vi "VisionMain.vi"(6 "Generated Distance Array":dbl[][](array[numeric]), 7 "Database Total Points":i32, 8 "Y Center":dbl, 9 "X Center":dbl, 10 "Original Plots":T1(array[cluster]), 11 "Plots Captured":T1(array[cluster])) -> (1 "alpha":dbl, 2 "dy":dbl, 3 "dx":dbl)   [LabVIEW 2012]
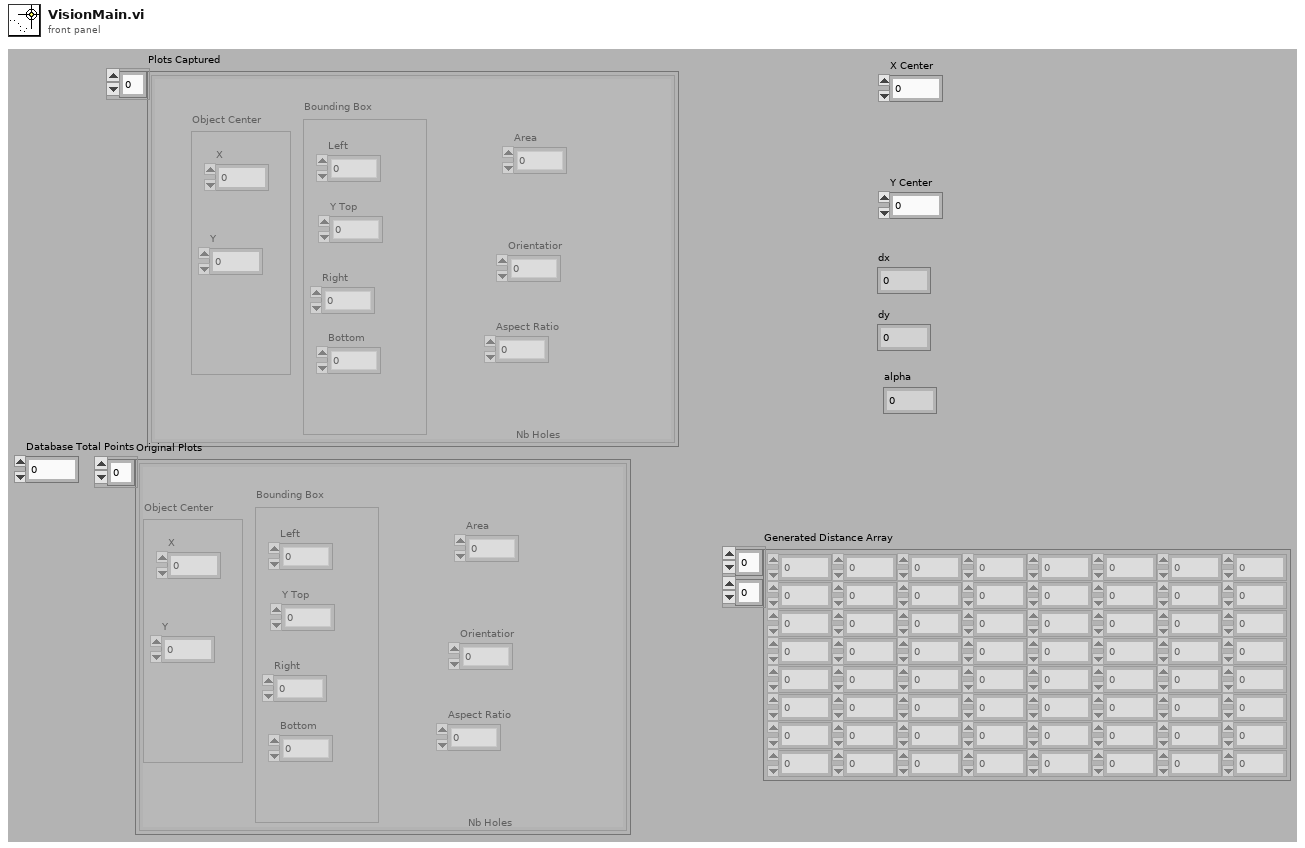
[diagram p1: front panel]
types:
  T1 = cluster{"Object Center":cluster{"X":dbl, "Y":dbl}, "Bounding Box":cluster{"Left":dbl, "Right":dbl, "Bottom":dbl, "Y Top":dbl}, "Area":dbl, "Orientatior":dbl, "Aspect Ratio":dbl, "Nb Holes":dbl}[]
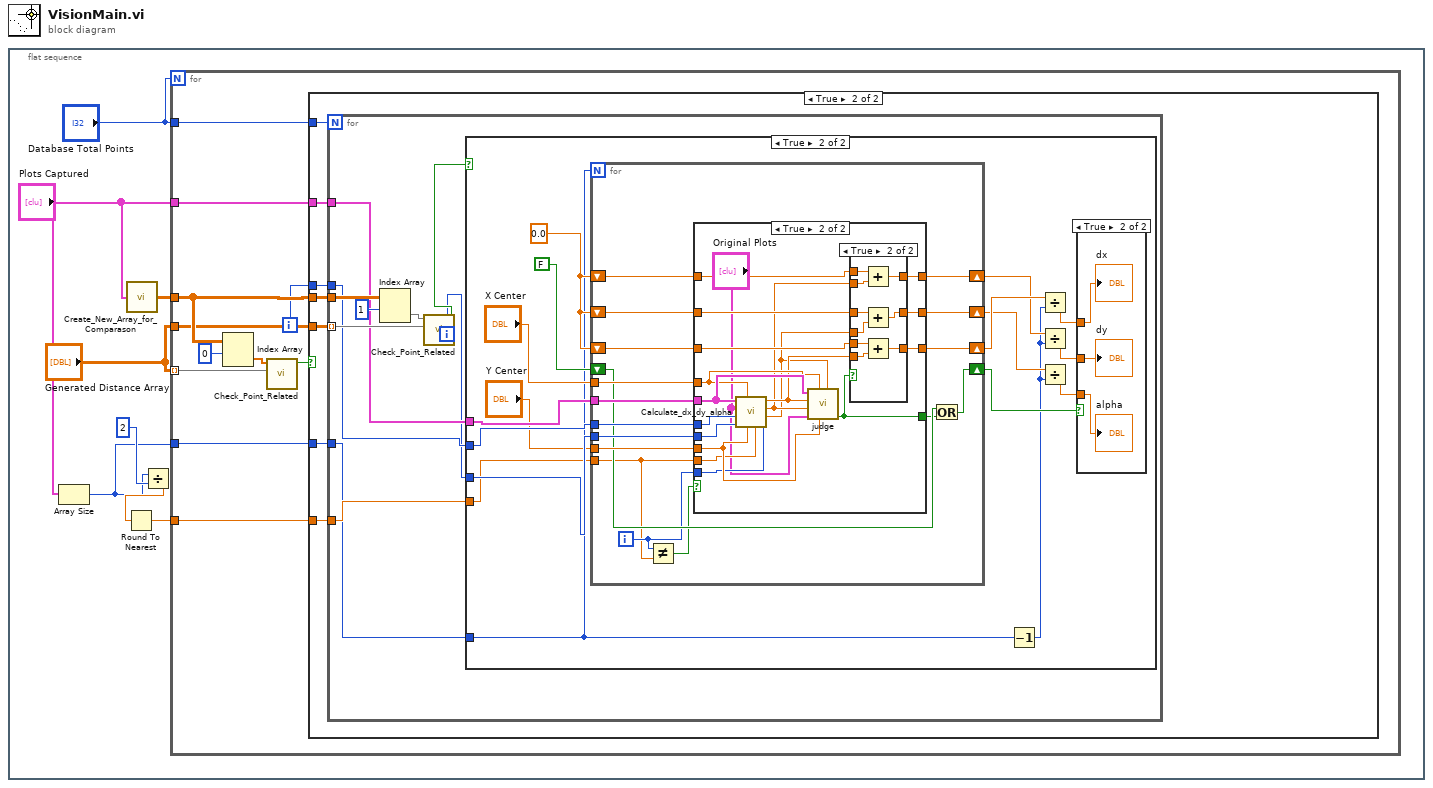
[diagram p0: block diagram]
diagram:
  n1 = flat-sequence {
    frame #0 {
      n2 = Array Size(array="Plots Captured") -> (size(s)=w2:i32)
      n3 = call "Create_New_Array_for_Comparason.vi"("Captured Plots"="Plots Captured") -> ("Generated Distance Array"=w8:dbl[][])
      n4 = Divide(x=w2, y=2) -> (x/y=w4:dbl)
      n5 = Round To Nearest(number=w4) -> (nearest integer value=w3:dbl)
      n6 = for {
        N: "Database Total Points" -> [_]
        tunnel: w8 -> [w16]
        tunnel: "Generated Distance Array" -> [w15] mode=indexing
        tunnel: "Generated Distance Array" -> [w14]
        tunnel: "Plots Captured" -> [w13]
        tunnel: "Database Total Points" -> [w11]
        tunnel: w3 -> [w10]
        tunnel: w2 -> [w9]
        i -> [w12]
        n7 = Index Array(array=w16, index (row)=0) -> (element=w18:dbl[])  [unwired: 1 in]
        n8 = call "Check_Point_Related.vi"("Original Plots"=w15, "Captured Plots"=w18) -> ("result"=w17:bool)  [unwired: 9 in]
        n9 = case shown="True" w17 {
          tunnel: w16 -> [_ w26]
          tunnel: w14 -> [_ w25]
          tunnel: w13 -> [_ w24]
          tunnel: w12 -> [_ w23]
          tunnel: w11 -> [_ w22]
          tunnel: w10 -> [_ w21]
          tunnel: w9 -> [_ w20]
          frame False {
          }
          frame True {
            n10 = for {
              N: w22 -> [_]
              tunnel: w26 -> [w36]
              tunnel: w25 -> [w32] mode=indexing
              tunnel: w24 -> [w31]
              tunnel: w23 -> [w30]
              tunnel: w21 -> [w28]
              tunnel: w20 -> [w27]
              i -> [w29]
              n11 = Index Array(array=w36, index (row)=1) -> (element=w34:dbl[])  [unwired: 1 in]
              n12 = call "Check_Point_Related.vi"("Original Plots"=w32, "Captured Plots"=w34) -> ("result"=w33:bool)  [unwired: 9 in]
              n13 = case shown="True" w33 {
                tunnel: w31 -> [_ w51]
                tunnel: w30 -> [_ w53]
                tunnel: w29 -> [_ w52]
                tunnel: w28 -> [_ w48]
                tunnel: w27 -> [_ w38]
                frame False {
                }
                frame True {
                  w47 = 0.0
                  n14 = for {
                    N: w38 -> [_]
                    tunnel: w53 -> [w70]
                    tunnel: w52 -> [w69]
                    tunnel: w51 -> [w68]
                    tunnel: "X Center" -> [w67]
                    tunnel: "Y Center" -> [w66]
                    tunnel: w48 -> [w55]
                    shift-right: [w62] -> w44
                    shift-left: w47 -> [w64]
                    shift-right: [w60] -> w42
                    shift-left: w47 -> [w63]
                    shift-right: [w61] -> w46
                    shift-left: w47 -> [w65]
                    shift-right: [w57] -> w39
                    shift-left: FALSE -> [w59]
                    i -> [w56]
                    n15 = Not Equal?(x=w56, y=w55) -> (x != y?=w54:bool)
                    n16 = case shown="True" w54 {
                      selector: w54 -> [w71 _]
                      tunnel: w70 -> [_ w92]
                      tunnel: w69 -> [_ w91]
                      tunnel: w68 -> [_ w90]
                      tunnel: w67 -> [_ w89]
                      tunnel: w66 -> [_ w88]
                      tunnel: w65 -> [w74 w87]
                      tunnel: w64 -> [w73 w86]
                      tunnel: w63 -> [w72 w85]
                      tunnel: [w73 w81] -> w62
                      tunnel: [w74 w80] -> w61
                      tunnel: [w72 w79] -> w60
                      tunnel: [w71 w78] -> w58
                      tunnel: w56 -> [_ w77]
                      tunnel: w55 -> [_ w76]
                      frame False {
                      }
                      frame True {
                        n17 = call "Calculate_dx_dy_alpha.vi"("index 2"=w77, "index 1"=w76, "c_y"=w88, "c_x"=w89, "Corresponding Point #2"=w91, "Corresponding Point #1"=w92, "Original Plots"="Original Plots", "Captured Plots"=w90) -> ("alpha"=w82:dbl, "dy"=w83:dbl, "dx"=w84:dbl)  [unwired: 1 in]
                        n18 = call "judge.vi"("alpha"=w82, "c_y"=w88, "c_x"=w89, "Original Plots"="Original Plots", "dy"=w83, "dx"=w84, "Captured Plots"=w90) -> ("result"=w78:bool)  [unwired: 4 in]
                        n19 = case shown="True" w78 {
                          tunnel: w87 -> [w95 w104]
                          tunnel: w86 -> [w94 w103]
                          tunnel: w85 -> [w93 w102]
                          tunnel: w84 -> [_ w101]
                          tunnel: w83 -> [_ w100]
                          tunnel: w82 -> [_ w99]
                          tunnel: [w95 w98] -> w80
                          tunnel: [w94 w97] -> w81
                          tunnel: [w93 w96] -> w79
                          frame False {
                          }
                          frame True {
                            n20 = Add(x=w103, y=w100) -> (x+y=w97:dbl)
                            n21 = Add(x=w102, y=w99) -> (x+y=w96:dbl)
                            n22 = Add(x=w104, y=w101) -> (x+y=w98:dbl)
                          }
                        }
                      }
                    }
                    n23 = Or(x=w59, y=w58) -> (x .or. y?=w57:bool)
                  }
                  n24 = Decrement(x=w38) -> (x-1=w37:i32)
                  n25 = Divide(x=w46, y=w37) -> (x/y=w45:dbl)
                  n26 = Divide(x=w44, y=w37) -> (x/y=w43:dbl)
                  n27 = Divide(x=w42, y=w37) -> (x/y=w41:dbl)
                  n28 = case shown="True" w39 {
                    tunnel: w45 -> [_ w107]
                    tunnel: w43 -> [_ w106]
                    tunnel: w41 -> [_ w105]
                    frame False {
                    }
                    frame True {
                      "dx" <- w107
                      "dy" <- w106
                      "alpha" <- w105
                    }
                  }
                }
              }
            }
          }
        }
      }
    }
  }
